vi "Get Interface Names from Resource Array.vi"(11 "fpga resources":T1[](array[typedef]) {"fpga cd" format="%.0x"}) -> (2 "Interface Names":string[](array[string]), 3 "fpga resources out":T1[](array[typedef]) {"fpga cd" format="%.0x"})   [LabVIEW 2016, in "FPGA RM System Definition API.lvlib"]
uses:
  FPGA RM System Definition API.lvlib
  Types/resources.ctl
  <vilib>/NI Veristand/Custom Device API/Custom Device Item Ref.ctl
  Shared/Types/fpga resource.ctl
  Shared/Types/Channel Type.ctl
  <vilib>/NI VeriStand/Custom Device API/Custom Device API.lvlib
  Shared/FPGA RM Shared API.lvlib
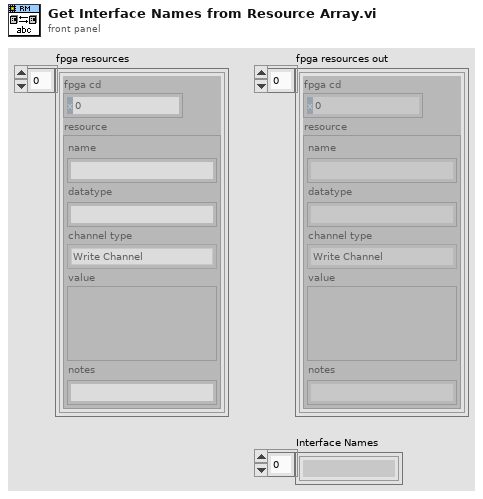
[diagram p1: front panel]
types:
  T1 = typedef "FPGA RM System Definition API.lvlib/resources.ctl" = cluster{"fpga cd":T2, "resource":T3}
  T2 = typedef "Custom Device API.lvlib/Custom Device Item Ref.ctl" = u64
  T3 = typedef "FPGA RM Shared API.lvlib/fpga resource.ctl" = cluster{"name":string, "datatype":string, "channel type":T4, "value":variant, "notes":string}
  T4 = typedef "FPGA RM Shared API.lvlib/Channel Type.ctl" = enum16{"Write Channel", "Read Channel", "Write Waveform", "Read Waveform"}
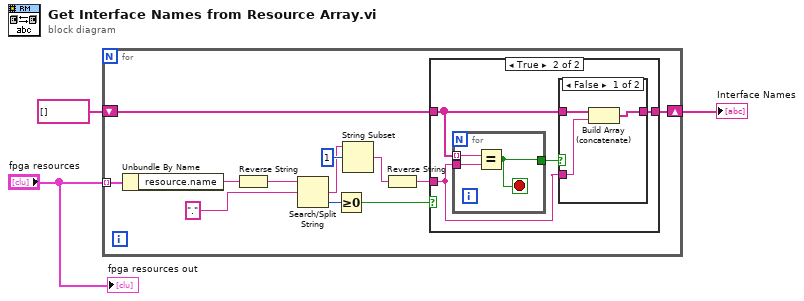
[diagram p0: block diagram]
diagram:
  n1 = for {
    tunnel: "fpga resources" -> [w15] mode=indexing
    shift-right: [w10] -> w3
    shift-left: string[] [] -> [w13]
    n2 = Unbundle By Name(w15) -> ("resource.name"=w9:string)
    n3 = Reverse String(1:w9) -> (0:w8:string)
    n4 = Search/Split String(string=w8, search string/char (-)=".") -> (match + rest of string=w4:string, offset of match=w12:i32)  [unwired: 1 in, 1 out]
    n5 = Greater Or Equal To 0?(x=w12) -> (x >= 0?=w11:bool)
    n6 = String Subset(string=w4, offset (0)=1) -> (substring=w6:string)  [unwired: 1 in]
    n7 = Reverse String(1:w6) -> (0:w5:string)
    n8 = case shown="True" w11 {
      tunnel: w13 -> [w16 w19]
      tunnel: w5 -> [_ w18]
      tunnel: [w16 w17] -> w10
      frame False {
      }
      frame True {
        n9 = for {
          tunnel: w19 -> [w27] mode=indexing
          tunnel: w18 -> [w25]
          tunnel: [w26] -> w20
          stop <- w26 stop-if-true
          n10 = Equal?(x=w27, y=w25) -> (x = y?=w26:bool)
        }
        n11 = case shown="False" w20 {
          tunnel: w19 -> [w23 w24]
          tunnel: w18 -> [w22 _]
          tunnel: [w21 w24] -> w17
          frame False {
            n12 = Build Array (concatenate)(w23, w22) -> (w21:string[])
          }
          frame True {
          }
        }
      }
    }
  }
  "Interface Names" <- w3
  "fpga resources out" <- "fpga resources"
